vi "uTTA_ScaleMeasurementData.vi"(7 "Filter Signals":bool, 8 "uTTA_MetaData_in":T3 {"No Suspect Lines" format="%.3pV"; "Interpolation Factor m" format="%.2g"; "Interpolation Offset" format="%.2g"; "Chip Size" format="%.2gmm²"; "Heating Power" format="%.3pW"; "Cool Volt Deviation" format="%.3pV"; "Cool Voltage" format="%.3pV"}, 9 "uTTA_MeasureData":T1, 11 "CAL_File":path) -> (1 "MeasData_out":T2, 3 "Graph_out":cluster{"Array":dbl[], "Array":dbl[]}[](array[cluster]), 4 "RunTime Scale":dbl)   [LabVIEW 2021]
uses:
  uTTA_MetaData.ctl
  CTL_uTTA_MeasurementData.ctl
  CTL_uTTA_MeasurementDataValues.ctl
  <vilib>/Analysis/3filter.llb/Filter Passband Type.ctl
  <vilib>/ptbypt/NI_PtbyPt.lvlib
  <vilib>/Analysis/NI_AALBase.lvlib
panel:
  out "F_Filter":dbl
  out "Fs":dbl
  in  "Filter Freq":dbl=10.0 format="%#_13g"
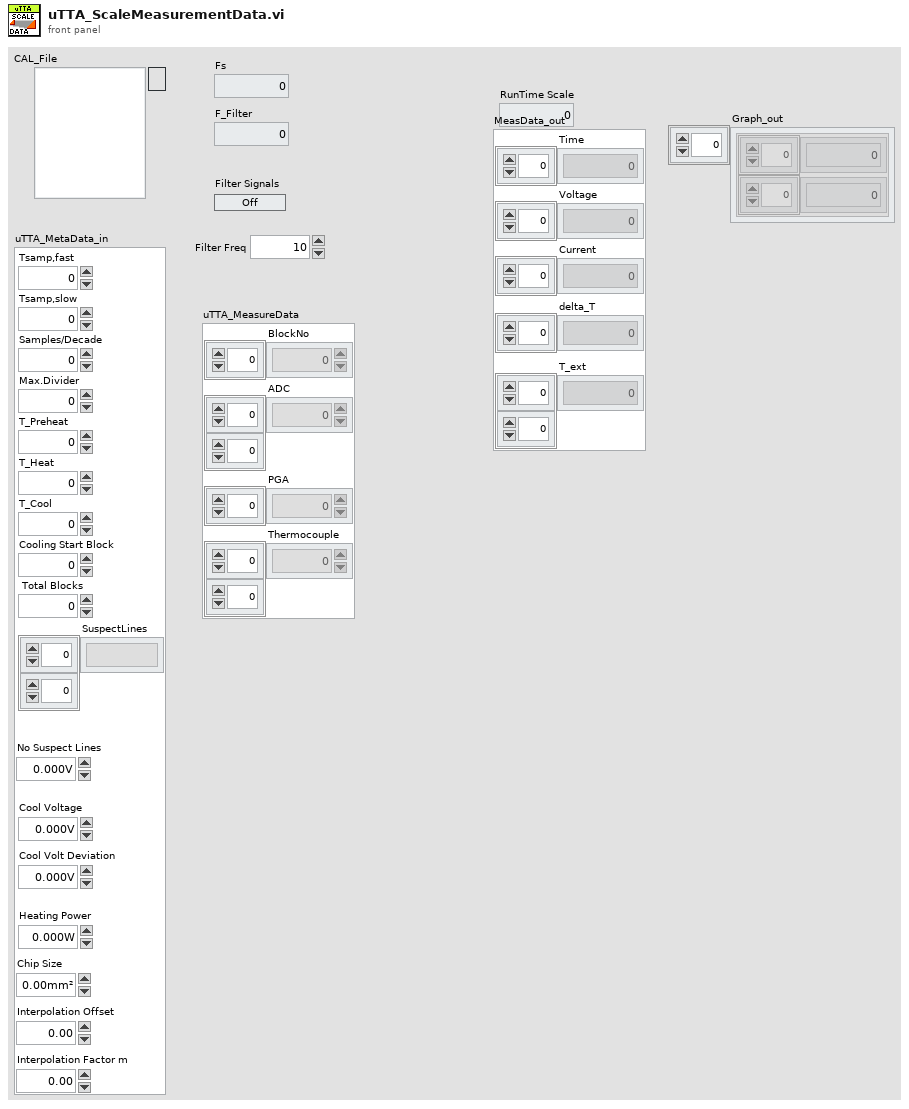
[diagram p1: front panel]
types:
  T1 = typedef "CTL_uTTA_MeasurementDataValues.ctl" = cluster{"BlockNo":i32[], "ADC":i32[][], "PGA":i32[], "Thermocouple":dbl[][]}
  T2 = typedef "CTL_uTTA_MeasurementData.ctl" = cluster{"Time":dbl[], "Voltage":dbl[], "Current":dbl[], "delta_T":dbl[], "T_ext":dbl[][]}
  T3 = typedef "uTTA_MetaData.ctl" = cluster{"Tsamp,fast":dbl, "Tsamp,slow":dbl, "Samples/Decade":u32, "Max.Divider":u32, "T_Preheat":dbl, "T_Heat":dbl, "T_Cool":dbl, "Cooling Start Block":u32, " Total Blocks":u32, "SuspectLines":string[][], "Cool Voltage":dbl, "Cool Volt Deviation":dbl, "Heating Power":dbl, "Chip Size":dbl, "Interpolation Offset":dbl, "Interpolation Factor m":dbl, "No Suspect Lines":u32}
  T4 = typedef "NI_AALBase.lvlib/Filter Passband Type.ctl" = enum32{"Lowpass", "Highpass", "Bandpass", "Bandstop"}
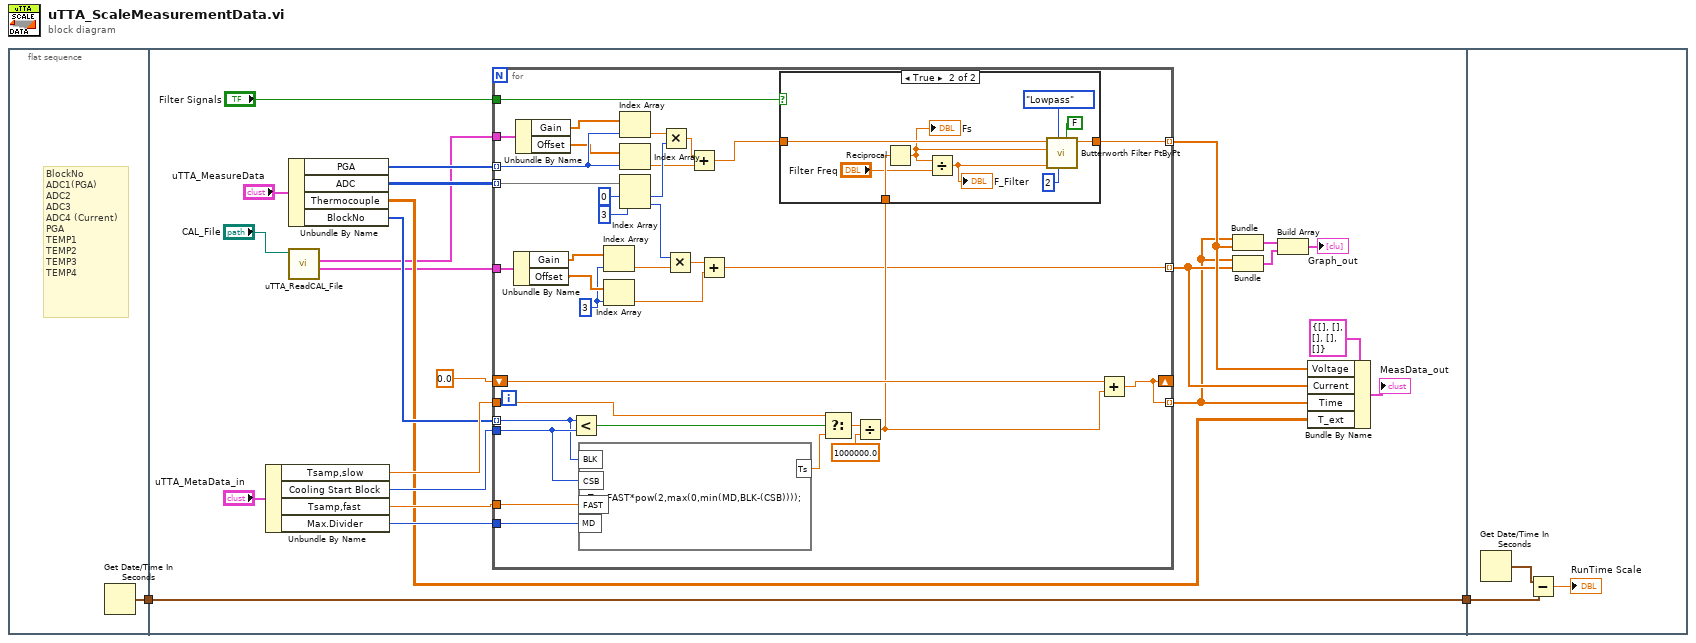
[diagram p0: block diagram]
diagram:
  n1 = flat-sequence {
    tunnel: [w3] -> w1
    tunnel: [w19] -> w2
    tunnel: w1 -> [w19]
    tunnel: w2 -> [w75]
    frame #0 {
      # "BlockNo\nADC1(PGA)\nADC2\nADC3\nADC4 (Current)\nPGA\nTEMP1\nTEMP2\nTEMP3\nTEMP4"
      n2 = Get Date/Time In Seconds() -> (seconds since 1Jan1904=w3:timestamp)
    }
    frame #1 {
      n3 = Unbundle By Name("uTTA_MetaData_in") -> ("Tsamp,slow"=w22:dbl, "Cooling Start Block"=w23:u32, "Tsamp,fast"=w24:dbl, "Max.Divider"=w25:u32)
      n4 = Unbundle By Name("uTTA_MeasureData") -> ("PGA"=w9:i32[], "ADC"=w8:i32[][], "Thermocouple"=w6:dbl[][], "BlockNo"=w7:i32[])
      n5 = call "uTTA_ReadCAL_File.vi"("file path"="CAL_File") -> ("ADC"=w4:cluster{"Offset":dbl[], "Gain":dbl[]}, "PGA"=w5:cluster{"Offset":dbl[], "Gain":dbl[]})  [unwired: 8 in, 1 out]
      n6 = for {
        tunnel: w23 -> [w58]
        tunnel: w24 -> [w59]
        tunnel: w22 -> [w60]
        shift-right: [w53] -> _
        shift-left: 0.0 ("default (0 DBL)") -> [w61]
        tunnel: w25 -> [w57]
        tunnel: [w53] -> w13 mode=indexing
        tunnel: [w49] -> w15 mode=indexing
        tunnel: [w46] -> w14 mode=indexing
        tunnel: "Filter Signals" -> [w47]
        tunnel: w9 -> [w45] mode=indexing
        tunnel: w8 -> [w44] mode=indexing
        tunnel: w7 -> [w39] mode=indexing
        tunnel: w5 -> [w38]
        tunnel: w4 -> [w33]
        w29 = 3 ("index")
        n7 = Unbundle By Name(w33) -> ("Gain"=w32:dbl[], "Offset"=w30:dbl[])
        n8 = Unbundle By Name(w38) -> ("Gain"=w36:dbl[], "Offset"=w37:dbl[])
        n9 = Less?(x=w39, y=w58) -> (x < y?=w62:bool)
        n10 = formula code="Ts=FAST*pow(2,max(0,min(MD,BLK-(CSB))));"("CSB"=w58, "BLK"=w39, "FAST"=w59, "MD"=w57) -> ("Ts"=w56:dbl)
        n11 = Index Array(array=w32, index=w29) -> (element=w31:dbl)
        n12 = Index Array(array=w30, index=w29) -> (element=w28:dbl)
        n13 = Index Array(array=w36, index=w45) -> (element=w35:dbl)
        n14 = Index Array(array=w37, index=w45) -> (element=w34:dbl)
        n15 = Index Array(array=w44, index #1=0 ("index"), index #2=3 ("index")) -> (element #1=w41:i32, element #2=w40:i32)
        n16 = Multiply(x=w35, y=w41) -> (x*y=w52:dbl)
        n17 = Multiply(x=w40, y=w31) -> (x*y=w51:dbl)
        n18 = Add(x=w52, y=w34) -> (x+y=w50:dbl)
        n19 = Add(x=w51, y=w28) -> (x+y=w46:dbl)
        n20 = Select(t=w60, s=w62, f=w56) -> (s? t:f=w55:dbl)
        n21 = Divide(x=w55, y=1000000.0) -> (x/y=w48:dbl)
        n22 = case shown="True" w47 {
          tunnel: w50 -> [w63 w72]
          tunnel: [w63 w71] -> w49
          tunnel: w48 -> [_ w70]
          frame False {
          }
          frame True {
            n23 = Reciprocal(x=w70) -> (1/x=w67:dbl)
            "Fs" <- w67
            n24 = Divide(x=w67, y="Filter Freq") -> (x/y=w66:dbl)
            "F_Filter" <- w66
            n25 = call <vilib>:"Butterworth Filter PtByPt.vi"("initialize"=FALSE, "order"=2, "filter type"=Filter_Passband_Type."Lowpass", "low cutoff freq: fl"=w66, "sampling freq: fs"=w67, "x"=w72) -> ("Filtered x"=w71:dbl)  [unwired: 3 in, 1 out]
          }
        }
        n26 = Add(x=w61, y=w48) -> (x+y=w53:dbl)
      }
      n27 = Bundle(w13, w15) -> (w18:cluster{dbl[], dbl[]})  [unwired: 1 in]
      n28 = Bundle(w13, w14) -> (w17:cluster{dbl[], dbl[]})  [unwired: 1 in]
      n29 = Build Array(w18, w17) -> (→"Graph_out":cluster{dbl[], dbl[]}[])
      n30 = Bundle By Name(cluster=T2 {"Time"=[], "Voltage"=[], "Current"=[], "delta_T"=[], "T_ext"=[]}, "Voltage"=w15, "Current"=w14, "Time"=w13, "T_ext"=w6) -> (→"MeasData_out":T2)
    }
    frame #2 {
      n31 = Get Date/Time In Seconds() -> (seconds since 1Jan1904=w74:timestamp)
      n32 = Subtract(x=w74, y=w75) -> (x-y=→"RunTime Scale":dbl)
    }
  }
